vi "noRepaetFileName(SubVI).vi"(1 "prompt overwrite?":bool, 3 "ext":string=".tdms", 4 "file name":string, 5 "subID":string, 6 "directory Path":path) -> (0 "file path out":path)   [LabVIEW 2011]
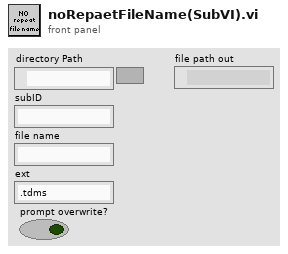
[diagram p1: front panel]
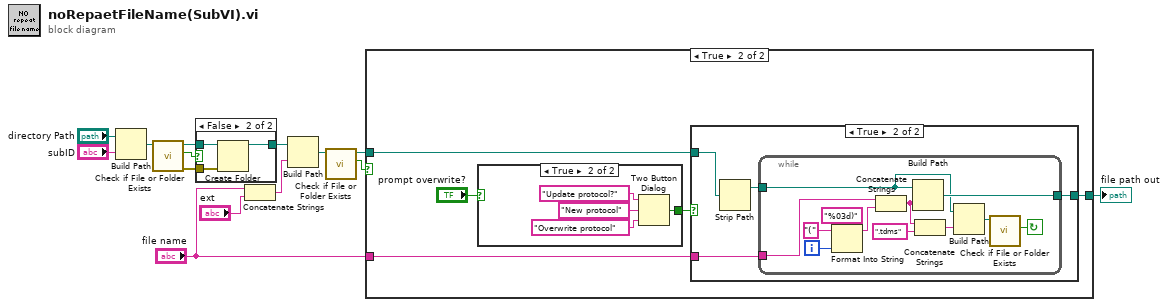
[diagram p0: block diagram]
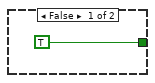
[diagram p3: hidden frame]
diagram:
  n1 = Build Path(base path="directory Path", name or relative path="subID") -> (appended path=w3:path)
  n2 = call <vilib>:"Check if File or Folder Exists.vi"("path"=w3) -> ("error out"=w5:errorcluster, "file or folder exists?"=w2:bool, "dup path"=w4:path)  [unwired: 8 in]
  n3 = case shown="False" w2 {
    tunnel: [w15 w18] -> w8
    tunnel: w4 -> [w15 w17]
    tunnel: w5 -> [_ w16]
    frame True {
    }
    frame False {
      n4 = Create Folder(path (use dialog)=w17, error in=w16) -> (created path=w18:path)  [unwired: 1 in, 2 out]
    }
  }
  n5 = Concatenate Strings("file name", "ext") -> (w11:string)
  n6 = Build Path(base path=w8, name or relative path=w11) -> (appended path=w7:path)
  n7 = call <vilib>:"Check if File or Folder Exists.vi"("path"=w7) -> ("file or folder exists?"=w10:bool, "dup path"=w9:path)  [unwired: 8 in, 1 out]
  n8 = case shown="True" w10 {
    tunnel: [w19 w24] -> w6
    tunnel: w9 -> [w19 w23]
    tunnel: "file name" -> [_ w22]
    frame False {
    }
    frame True {
      n9 = case shown="True" "prompt overwrite?" {
        tunnel: [TRUE ("T button?") w26] -> w21
        frame False {
        }
        frame True {
          n10 = Two Button Dialog(message="Update protocol?", 1:"Overwrite protocol" ("F button name (\"Cancel\")"), 2:"New protocol" ("T button name (\"OK\")")) -> (T button?=w26:bool)
        }
      }
      n11 = case shown="True" w21 {
        tunnel: [w30 w34] -> w24
        tunnel: w23 -> [w30 w33]
        tunnel: w22 -> [_ w31]
        frame False {
        }
        frame True {
          n12 = Strip Path(path=w33) -> (stripped path=w32:path)  [unwired: 1 out]
          n13 = while {
            tunnel: [w45] -> w34
            tunnel: w32 -> [w44]
            tunnel: w31 -> [w42]
            i -> [w43]
            stop <- w46 continue-if-true
            n14 = Format Into String(format string="%03d)", initial string="(", w43) -> (resulting string=w41:string)  [unwired: 1 in, 1 out]
            n15 = Concatenate Strings(w42, w41) -> (w37:string)
            n16 = Build Path(base path=w44, name or relative path=w37) -> (appended path=w45:path)
            n17 = Concatenate Strings(w37, ".tdms" ("string")) -> (w36:string)
            n18 = Build Path(base path=w44, name or relative path=w36) -> (appended path=w35:path)
            n19 = call <vilib>:"Check if File or Folder Exists.vi"("path"=w35) -> ("file or folder exists?"=w46:bool)  [unwired: 8 in, 2 out]
          }
        }
      }
    }
  }
  "file path out" <- w6
